vi "init add index to cluster.vi"(9 "dictionary index":i32, 10 "data cluster index":i32, 11 "data cluster in":T1[](array[typedef])) -> (3 "data cluster out":T1[](array[typedef]))   [LabVIEW 2013, in "Shared Memory runtime.lvclass"]
uses:
  Shared Memory runtime.lvclass
  channel runtime.ctl
  <vilib>/NI/Tag Bus Module Framework/channel/channel classification.ctl
  <vilib>/NI/Tag Bus/tag/Data Type.ctl
  <vilib>/NI/NI Linux RT IPC/Shared Memory/Classes/Shared Memory/Public/Controls/reference.ctl
  <vilib>/NI/NI Linux RT IPC/Shared Memory/Classes/Shared Memory/Shared Memory.lvclass
  <vilib>/NI/Tag Bus Module Framework/channel/TBM channel.lvclass
  <vilib>/NI/Tag Bus/tag/tag descriptor.lvclass
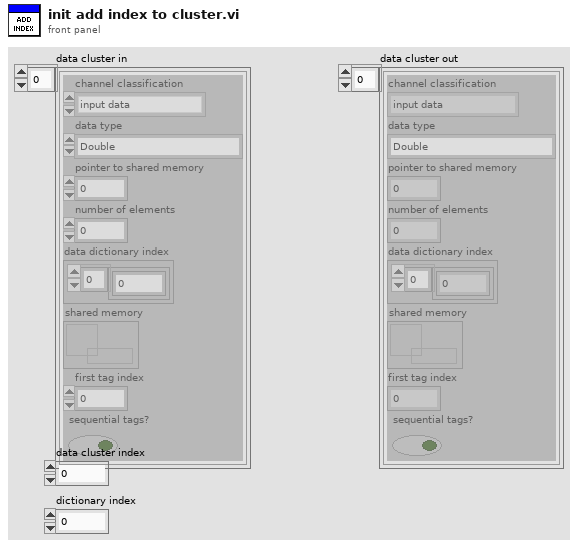
[diagram p1: front panel]
types:
  T1 = typedef "Shared Memory runtime.lvclass/channel runtime.ctl" = cluster{"channel classification":T2, "data type":T3, "pointer to shared memory":u64, "number of elements":u64, "data dictionary index":cluster{i32[]}, "shared memory":T4, "first tag index":i32, "sequential tags?":bool}
  T2 = typedef "TBM channel.lvclass/channel classification.ctl" = enum16{"input data", "output data", "processing parameter", "processing result"}
  T3 = typedef "tag bus.lvlib/tag descriptor.lvclass/Data Type.ctl" = enum16{"Double", "Single", "I64", "I32", "I16", "I8", "U64", "U32", "U16", "U8", "Boolean", "String", "Array of Double", "Array of Single", "Array of I64", "Array of I32", "Array of I16", "Array of I8", "Array of U64", "Array of U32", "Array of U16", "Array of U8", "Array of Boolean", "Array of String"}
  T4 = typedef "Shared Memory.lvlib/Shared Memory.lvclass/reference.ctl" = refnum<data-value>
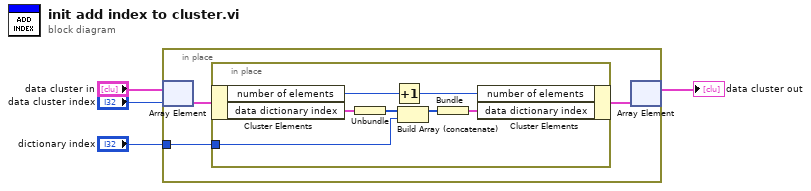
[diagram p0: block diagram]
diagram:
  n1 = in-place {
    in-place-border: "dictionary index" -> [w5]
    n2 = in-place-array #1("data cluster in", "data cluster index") -> (w7:T1)
    n3 = in-place {
      in-place-border: w5 -> [w8]
      n4 = in-place-cluster #2(w7) -> ("number of elements"=w14:u64, "data dictionary index"=w10:cluster{i32[]})
      n5 = Unbundle(w10) -> (w12:i32[])
      n6 = Increment(x=w14) -> (x+1=w13:u64)
      n7 = Build Array (concatenate)(w12, w8) -> (w11:i32[])
      n8 = Bundle(w11) -> (w9:cluster{i32[]})  [unwired: 1 in]
      n9 = in-place-cluster #2("number of elements"=w13, "data dictionary index"=w9) -> (w6:T1)
    }
    n10 = in-place-array #1(w6) -> (→"data cluster out":T1[])  [unwired: 1 out]
  }
